vi "Create String Times.vi"(8 "error in (no error)":errorcluster, 11 "Readout Charact in":refnum<class "Readout Charact.lvclass">) -> (0 "error out":errorcluster, 3 "Readout Charact out":refnum<class "Readout Charact.lvclass">)   [LabVIEW 2018, in "Readout Charact.lvclass"]
uses:
  Readout Charact.lvclass
  Readout Charact.lvclass/Readout Charact.ctl
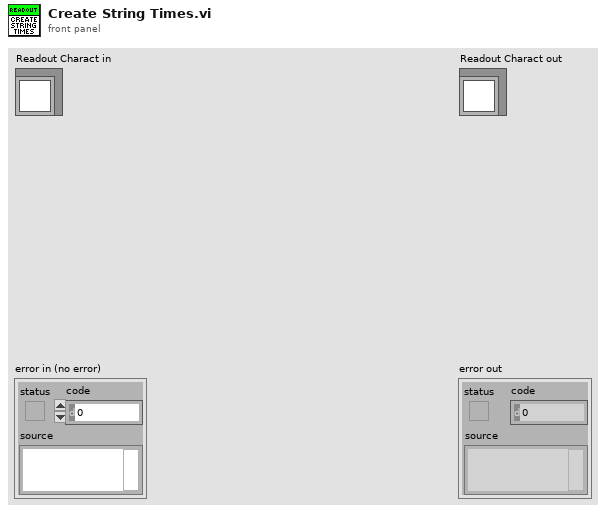
[diagram p1: front panel]
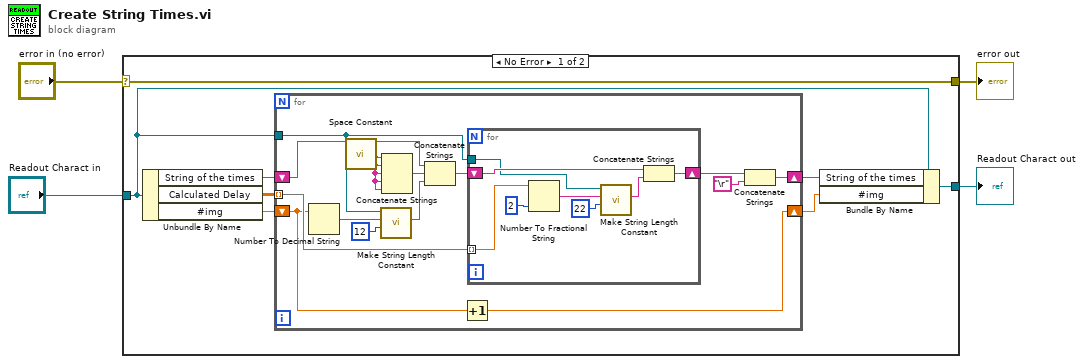
[diagram p0: block diagram]
diagram:
  n1 = case shown="No Error" "error in (no error)" {
    selector: "error in (no error)" -> [w12 w36]
    tunnel: [w12 w36] -> w3
    tunnel: [w10 w35] -> w1
    tunnel: "Readout Charact in" -> [w6 w35]
    frame No Error {
      n2 = Unbundle By Name(w6) -> ("String of the times"=w7:string, "Calculated Delay"=w5:dbl[][], "#img"=w9:dbl)
      n3 = for {
        tunnel: w6 -> [w15]
        shift-right: [w24] -> w11
        shift-left: w7 -> [w20]
        tunnel: w5 -> [w14] mode=indexing
        shift-right: [w23] -> w8
        shift-left: w9 -> [w13]
        n4 = Number To Decimal String(number=w13) -> (decimal integer string=w19:string)  [unwired: 1 in]
        n5 = call <vilib>:"Space Constant.vi"() -> ("String"=w18:string)
        n6 = call "Make String Length Constant.vi"("String Lenght"=i16 12 ("precision (6)"), "String in"=w19, "Readout Charact in"=w15) -> ("String out"=w16:string)  [unwired: 6 in, 2 out]
        n7 = Concatenate Strings(w18, w18, w18, w18, w18) -> (w17:string)
        n8 = Concatenate Strings(w20, w17, w16) -> (w21:string)
        n9 = Increment(x=w13) -> (x+1=w23:dbl)
        n10 = for {
          tunnel: w14 -> [w34] mode=indexing
          shift-right: [w29] -> w26
          shift-left: w21 -> [w30]
          tunnel: w15 -> [w28]
          n11 = Number To Fractional String(number=w34, precision (6)=i16 2) -> (F-format string=w32:string)  [unwired: 2 in]
          n12 = call "Make String Length Constant.vi"("String Lenght"=i16 22 ("precision (6)"), "String in"=w32, "Readout Charact in"=w28) -> ("String out"=w31:string)  [unwired: 6 in, 2 out]
          n13 = Concatenate Strings(w30, w31) -> (w29:string)
        }
        n14 = Concatenate Strings(w26, "\r") -> (w24:string)
      }
      n15 = Bundle By Name(cluster=w6, "String of the times"=w11, "#img"=w8) -> (w10:refnum<class "Readout Charact.lvclass">)
    }
    frame Error {
    }
  }
  "error out" <- w3
  "Readout Charact out" <- w1
